vi "DAQ6363_LoadHistGraph.vi"(8 "ErrIn(No Err)":errorcluster caption="entrée d'erreur (pas d'erreur)", 11 "Rate Mode":bool) -> (0 "ErrOut":errorcluster caption="sortie d'erreur", 1 "Graph":refnum<vi>, 2 "Dat":refnum<vi>, 3 "ViRef":refnum<vi>, 4 "MaxT ref":refnum<vi>, 5 "Avg ref":refnum<vi>, 6 "ClearRef":refnum<vi>)   [LabVIEW 2019]
panel:
  out "Exécution:État":T1(ring)
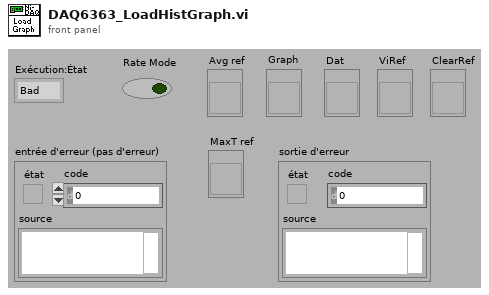
[diagram p1: front panel]
types:
  T1 = enum32{"Bad", "Idle", "Run top level", "Running"}
  T2 = enum8{"Enabled", "Disabled", "Disabled and Grayed Out"}
  T3 = enum32{"Invalid", "Standard", "Closed", "Hidden", "Minimized", "Maximized"}
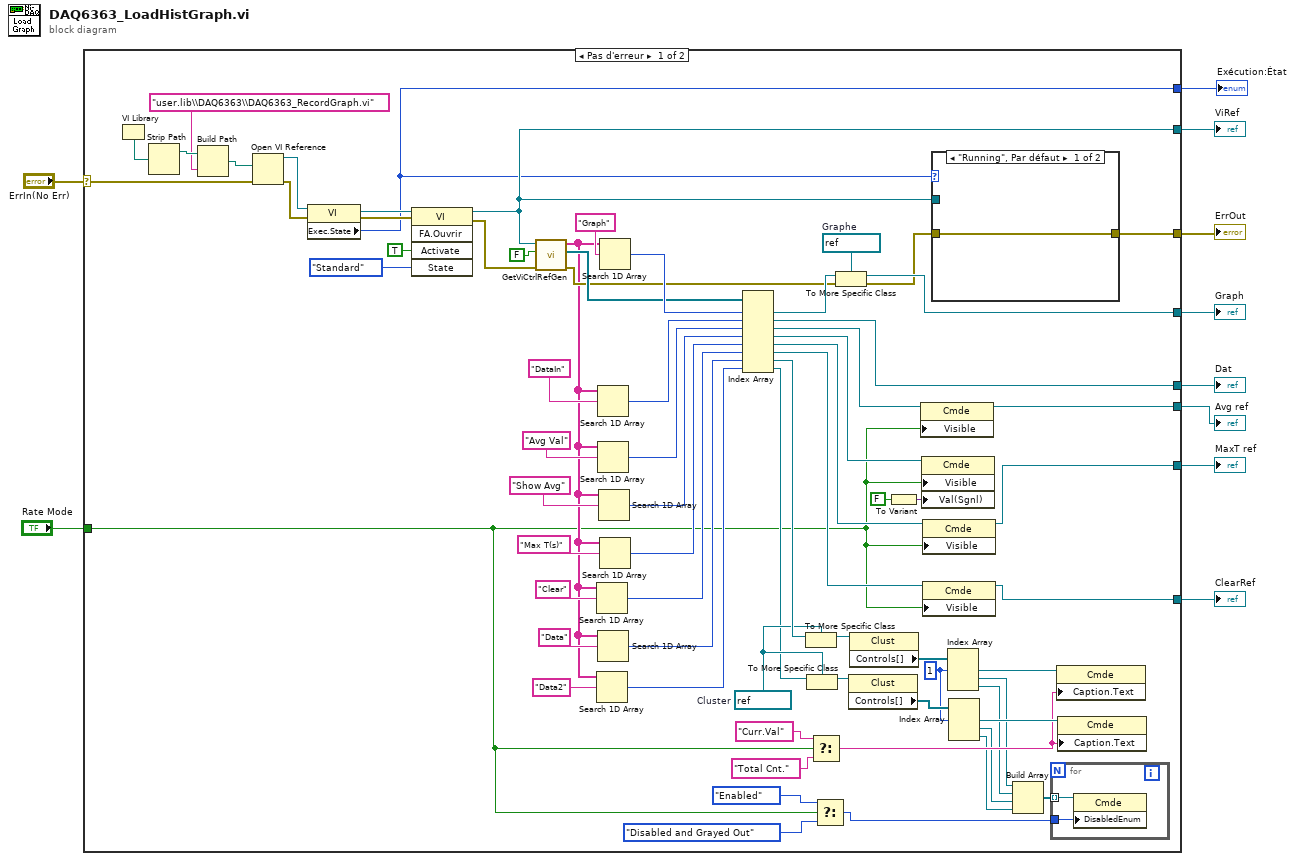
[diagram p0: block diagram]
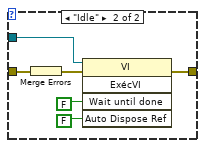
[diagram p2: hidden frame]
diagram:
  n1 = case shown="Pas d'erreur" "ErrIn(No Err)" {
    selector: "ErrIn(No Err)" -> [w68 w91]
    tunnel: [w74 w91] -> w9
    tunnel: [w77 _] -> w8
    tunnel: [w57 _] -> w7
    tunnel: [w56 _] -> w6
    tunnel: "Rate Mode" -> [w17 _]
    tunnel: [w48 _] -> w4
    tunnel: [w43 _] -> w3
    tunnel: [w39 _] -> w2
    tunnel: [w20 _] -> w1
    frame No Error {
      w27 = 1 ("indice")
      w32 = refnum<vi> refnum  # Cluster
      w76 = refnum<vi> refnum  # Graphe
      n2 = VI Library() -> (path=w69:path)
      n3 = Strip Path(path=w69) -> (stripped path=w62:path)  [unwired: 1 out]
      n4 = Build Path(base path=w62, name or relative path="user.lib\\DAQ6363\\DAQ6363_RecordGraph.vi" ("NomFichier")) -> (appended path=w61:path)
      n5 = Open VI Reference(vi path=w61, error in (no error)=w68) -> (vi reference=w66:refnum<vi>, error out=w65:errorcluster)  [unwired: 4 in]
      n6 = property class="VI"(reference=w66, error in=w65) -> (reference out=w63:refnum<vi>, error out=w64:errorcluster, "Exec.State"=w20:T1)
      n7 = invoke class="VI" method="FA.Ouvrir"(reference=w63, error in=w64, "Activate"=TRUE ("Activer ?"), "State"=T3."Standard" ("État")) -> (reference out=w56:refnum<vi>, error out=w67:errorcluster)  [unwired: 1 in, 3 out]
      n8 = call <userlib>:"GetViCtrlRefGen.vi"("ErrorIn(No Error)"=w67, "InclTabCTrl"=FALSE, "VIRef"=w56) -> ("sortie d'erreur"=w72:errorcluster, "ControlsRefs"=w73:refnum<vi>[], "ControlsNames"=w21:string[])  [unwired: 6 in]
      n9 = Search 1D Array(1D array=w21, element="Clear" ("élément")) -> (index of element=w41:i32)  [unwired: 1 in]
      n10 = Search 1D Array(1D array=w21, element="Data2" ("élément")) -> (index of element=w35:i32)  [unwired: 1 in]
      n11 = Search 1D Array(1D array=w21, element="DataIn" ("élément")) -> (index of element=w58:i32)  [unwired: 1 in]
      n12 = Search 1D Array(1D array=w21, element="Avg Val" ("élément")) -> (index of element=w51:i32)  [unwired: 1 in]
      n13 = Search 1D Array(1D array=w21, element="Data" ("élément")) -> (index of element=w36:i32)  [unwired: 1 in]
      n14 = Search 1D Array(1D array=w21, element="Show Avg" ("élément")) -> (index of element=w47:i32)  [unwired: 1 in]
      n15 = Search 1D Array(1D array=w21, element="Graph" ("élément")) -> (index of element=w79:i32)  [unwired: 1 in]
      n16 = Search 1D Array(1D array=w21, element="Max T(s)" ("élément")) -> (index of element=w45:i32)  [unwired: 1 in]
      n17 = Index Array(array=w73, index #1=w79, index #2=w58, index #3=w51, index #4=w47, index #5=w45, index #6=w41, index #7=w36, index #8=w35) -> (element #1=w78:refnum<vi>, element #2=w57:refnum<vi>, element #3=w53:refnum<vi>, element #4=w52:refnum<vi>, element #5=w44:refnum<vi>, element #6=w40:refnum<vi>, element #7=w34:refnum<vi>, element #8=w31:refnum<vi>)
      n18 = To More Specific Class(target class=w32, reference=w34) -> (specific class reference=w33:refnum<vi>)  [unwired: 1 in, 1 out]
      n19 = To More Specific Class(target class=w32, reference=w31) -> (specific class reference=w30:refnum<vi>)  [unwired: 1 in, 1 out]
      n20 = Select(t="Curr.Val" ("élément"), s=w17, f="Total Cnt." ("élément")) -> (s? t:f=w22:string)
      n21 = Select(t=T2."Enabled" ("Désactivé"), s=w17, f=T2."Disabled and Grayed Out" ("Désactivé")) -> (s? t:f=w11:T2)
      n22 = To More Specific Class(target class=w76, reference=w78, error in=w72) -> (specific class reference=w77:refnum<vi>, error out=w75:errorcluster)
      n23 = property class="Clust"(reference=w30) -> ("Controls[]"=w28:refnum<vi>[])  [unwired: 1 in, 2 out]
      n24 = property class="Clust"(reference=w33) -> ("Controls[]"=w29:refnum<vi>[])  [unwired: 1 in, 2 out]
      n25 = To Variant(anything=FALSE) -> (Variant=w50:variant)
      n26 = property class="Cmde"(reference=w53, "Visible"=w17) -> (reference out=w48:refnum<vi>)  [unwired: 1 in, 1 out]
      n27 = property class="Cmde"(reference=w52, "Visible"=w17, "Val(Sgnl)"=w50) -> ()  [unwired: 1 in, 2 out]
      n28 = property class="Cmde"(reference=w44, "Visible"=w17) -> (reference out=w43:refnum<vi>)  [unwired: 1 in, 1 out]
      n29 = property class="Cmde"(reference=w40, "Visible"=w17) -> (reference out=w39:refnum<vi>)  [unwired: 1 in, 1 out]
      n30 = case shown="\"Running\", Par défaut" w20 {
        tunnel: w75 -> [w84 w88]
        tunnel: [w84 w86] -> w74
        tunnel: w56 -> [_ w85]
        frame "Running", Default {
        }
        frame "Idle" {
          n31 = Merge Errors(w88) -> (w87:errorcluster)
          n32 = invoke class="VI" method="ExécVI"(reference=w85, error in=w87, "Wait until done"=FALSE ("Attendre la fin"), "Auto Dispose Ref"=FALSE ("Supprimer la référence automatiquement")) -> (error out=w86:errorcluster)  [unwired: 1 in, 4 out]
        }
      }
      n33 = Index Array(array=w29, index #1=w27) -> (element #1=w26:refnum<vi>, element #2=w16:refnum<vi>, element #3=w15:refnum<vi>)  [unwired: 2 in]
      n34 = Index Array(array=w28, index #1=w27) -> (element #1=w25:refnum<vi>, element #2=w14:refnum<vi>, element #3=w13:refnum<vi>)  [unwired: 2 in]
      n35 = Build Array(w16, w15, w14, w13) -> (w12:refnum<vi>[])
      n36 = for {
        tunnel: w12 -> [w83] mode=indexing
        tunnel: w11 -> [w82]
        n37 = property class="Cmde"(reference=w83, "DisabledEnum"=w82) -> ()  [unwired: 1 in, 2 out]
      }
      n38 = property class="Cmde"(reference=w26, "Caption.Text"=w22) -> ()  [unwired: 1 in, 2 out]
      n39 = property class="Cmde"(reference=w25, "Caption.Text"=w22) -> ()  [unwired: 1 in, 2 out]
    }
    frame Error {
    }
  }
  "ErrOut" <- w9
  "Graph" <- w8
  "Dat" <- w7
  "ViRef" <- w6
  "Avg ref" <- w4
  "MaxT ref" <- w3
  "ClearRef" <- w2
  "Exécution:État" <- w1
